vi "HandleTab.vi"(6 "Forward?":bool=TRUE, 8 "error in (no error)":errorcluster, 11 "TabbedControls":T1[](array[typedef])) -> (0 "error out":errorcluster, 3 "Discard?":bool)   [LabVIEW 2017, in "ContextHelpEditor.lvlib"]
uses:
  ContextHelpEditor.lvlib
  TabbedControl--cluster.ctl
  TabChange State--cluster.ctl
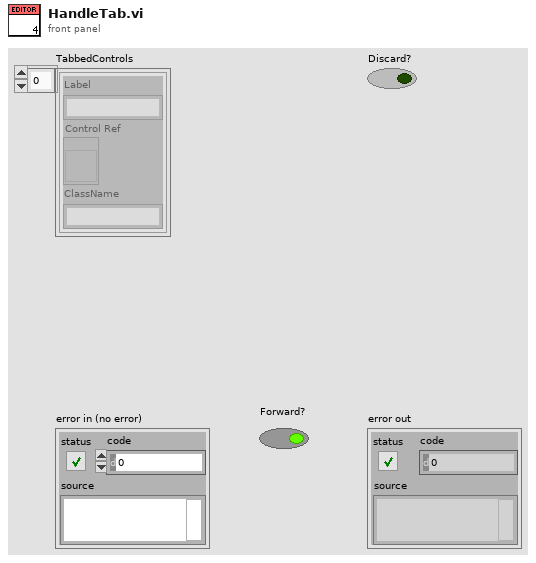
[diagram p1: front panel]
types:
  T1 = typedef "ContextHelpEditor.lvlib/TabbedControl--cluster.ctl" = cluster{"Label":string, "Control Ref":refnum<vi>, "ClassName":string}
  T2 = typedef "ContextHelpEditor.lvlib/TabChange State--cluster.ctl" = enum16{"CHECK_CURRENT_TYPE", "CHECK_PREVIOUS_TYPE", "CHECK_NEXT_TYPE", "CHECK_JUMP_INNER_MCLISTBOX", "JUMP_CURRENT_FW_MCLISTBOX", "JUMP_CURRENT_BACK_MCLISTBOX", "ACTIVATE_FIRST_ELEM_MCLISTBOX", "ACTIVATE_LAST_ELEM_MCLISTBOX", "ACTIVATE_NEXT_CONTROL", "ACTIVATE_PREV_CONTROL"}
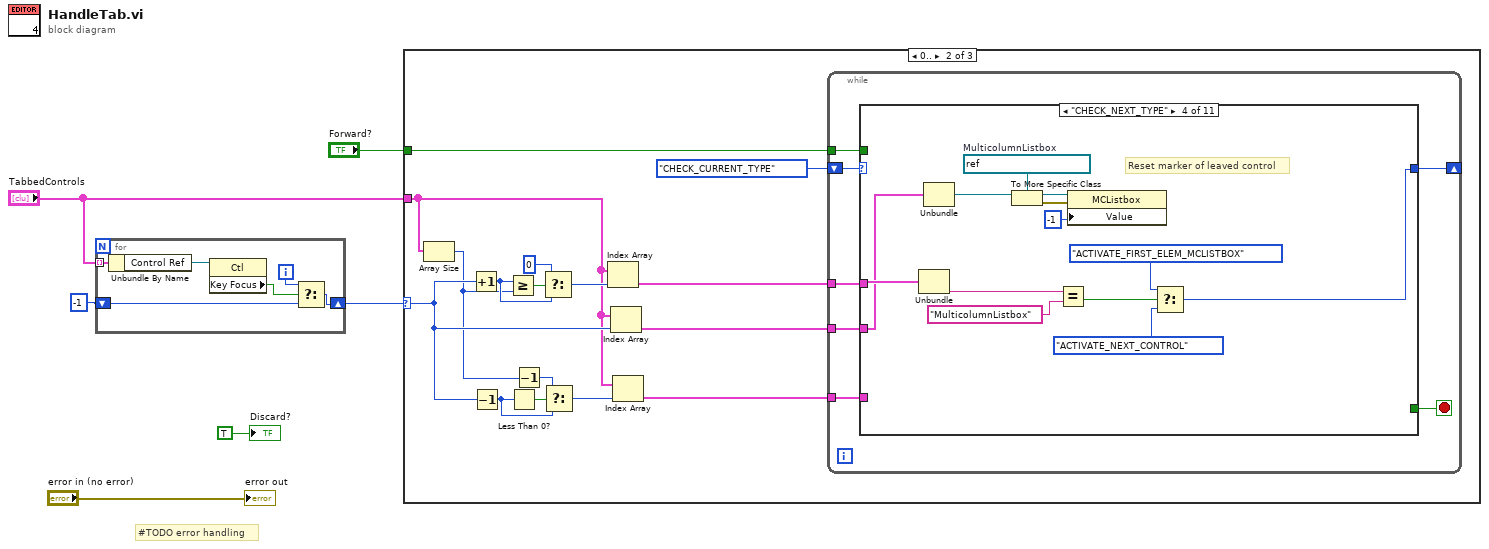
[diagram p0: block diagram]
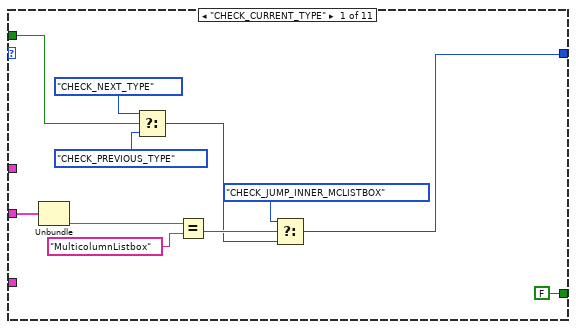
[diagram p3: hidden frame]
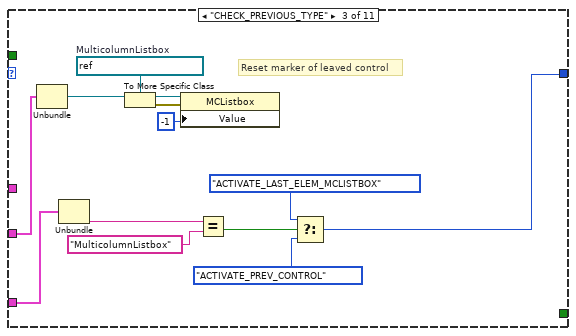
[diagram p5: hidden frame]
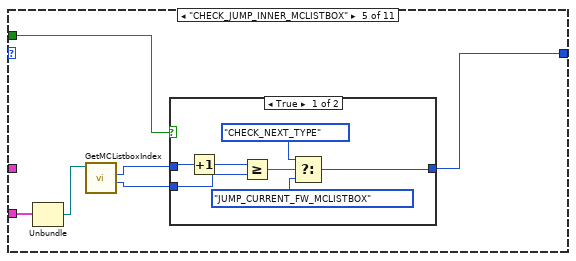
[diagram p6: hidden frame]
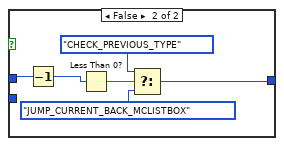
[diagram p7: hidden frame]
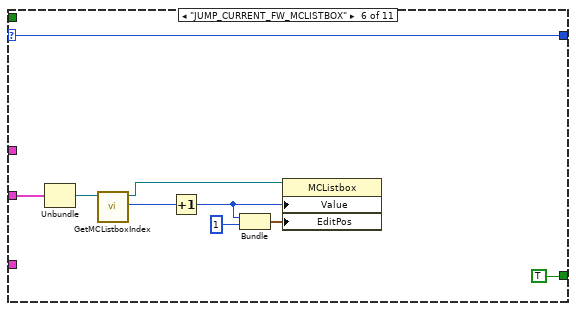
[diagram p8: hidden frame]
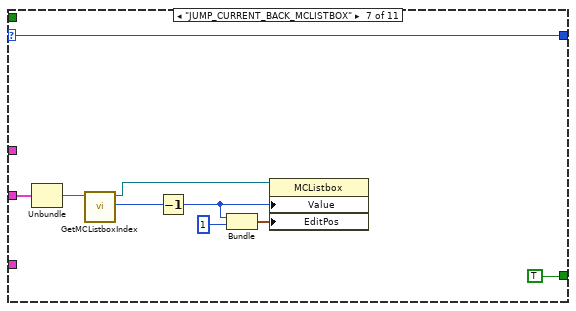
[diagram p9: hidden frame]
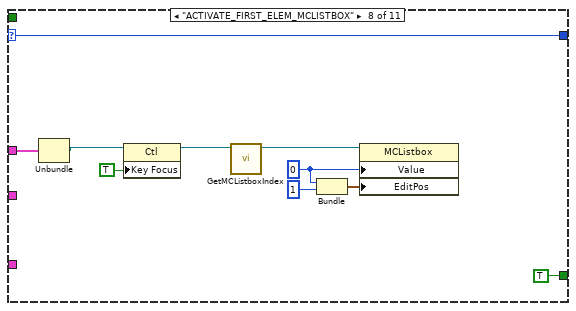
[diagram p10: hidden frame]
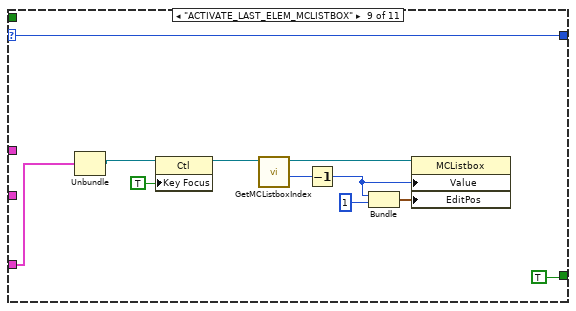
[diagram p11: hidden frame]
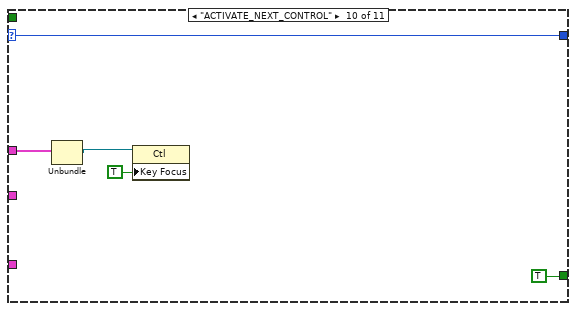
[diagram p12: hidden frame]
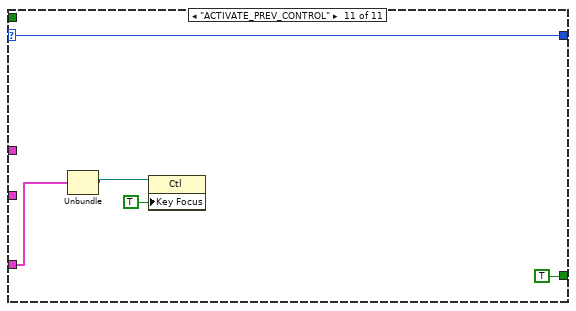
[diagram p13: hidden frame]
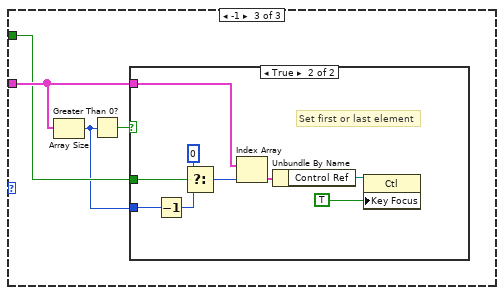
[diagram p14: hidden frame]
diagram:
  # "#TODO error handling"
  n1 = for {
    tunnel: "TabbedControls" -> [w12] mode=indexing
    shift-right: [w10] -> w3
    shift-left: -1 -> [w7]
    i -> [w8]
    n2 = Unbundle By Name(w12) -> ("Control Ref"=w11:refnum<vi>)
    n3 = property class="Ctl"(reference=w11) -> ("Key Focus"=w9:bool)  [unwired: 1 in, 2 out]
    n4 = Select(t=w8, s=w9, f=w7) -> (s? t:f=w10:i32)
  }
  n5 = case shown="0.." w3 {
    selector: w3 -> [_ w23 _]
    tunnel: "TabbedControls" -> [_ w19 w145]
    tunnel: "Forward?" -> [_ w16 w143]
    frame Default {
    }
    frame 0.. {
      n6 = Array Size(array=w19) -> (size(s)=w21:i32)
      n7 = Increment(x=w23) -> (x+1=w25:i32)
      n8 = Decrement(x=w23) -> (x-1=w22:i32)
      n9 = Greater Or Equal?(x=w25, y=w21) -> (x >= y?=w28:bool)
      n10 = Less Than 0?(x=w22) -> (x < 0?=w24:bool)
      n11 = Decrement(x=w21) -> (x-1=w20:i32)
      n12 = Select(t=0, s=w28, f=w25) -> (s? t:f=w26:i32)
      n13 = Select(t=w20, s=w24, f=w22) -> (s? t:f=w18:i32)
      n14 = Index Array(array=w19, index=w26) -> (element=w15:T1)
      n15 = Index Array(array=w19, index=w23) -> (element=w14:T1)
      n16 = Index Array(array=w19, index=w18) -> (element=w13:T1)
      n17 = while {
        shift-right: [w34] -> _
        shift-left: TabChange_State--cluster."CHECK_CURRENT_TYPE" -> [w35]
        tunnel: w16 -> [w33]
        tunnel: w15 -> [w31]
        tunnel: w14 -> [w30]
        tunnel: w13 -> [w29]
        stop <- w32 stop-if-true
        n18 = case shown="\"CHECK_NEXT_TYPE\"" w35 {
          selector: w35 -> [_ w47 _ _ _ w93 w102 w113 w121 w132 w137]
          tunnel: [w37 w47 w54 w67 w76 w93 w102 w113 w121 w132 w137] -> w34
          tunnel: w33 -> [w42 _ _ _ w77 _ _ _ _ _ _]
          tunnel: [FALSE _ _ _ _ TRUE TRUE TRUE TRUE TRUE TRUE] -> w32
          tunnel: w31 -> [_ _ _ w70 _ _ _ w117 _ w134 _]
          tunnel: w30 -> [w45 _ w51 w61 w79 w100 w104 _ _ _ _]
          tunnel: w29 -> [_ _ w55 _ _ _ _ _ w127 _ w139]
          frame "CHECK_CURRENT_TYPE" {
            n19 = Unbundle(w45) -> ("ClassName"=w44:string)  [unwired: 2 out]
            n20 = Select(t=TabChange_State--cluster."CHECK_NEXT_TYPE", s=w42, f=TabChange_State--cluster."CHECK_PREVIOUS_TYPE") -> (s? t:f=w38:T2)
            n21 = Equal?(x=w44, y="MulticolumnListbox") -> (x = y?=w39:bool)
            n22 = Select(t=TabChange_State--cluster."CHECK_JUMP_INNER_MCLISTBOX", s=w39, f=w38) -> (s? t:f=w37:T2)
          }
          frame Default {
          }
          frame "CHECK_PREVIOUS_TYPE" {
            w48 = refnum<vi> refnum  # MulticolumnListbox
            # "Reset marker of leaved control"
            n23 = Unbundle(w51) -> ("Control Ref"=w52:refnum<vi>)  [unwired: 2 out]
            n24 = Unbundle(w55) -> ("ClassName"=w60:string)  [unwired: 2 out]
            n25 = To More Specific Class(target class=w48, reference=w52) -> (specific class reference=w49:refnum<vi>, error out=w50:errorcluster)  [unwired: 1 in]
            n26 = property class="MCListbox"(reference=w49, error in=w50, "Value"=-1) -> ()  [unwired: 2 out]
            n27 = Equal?(x=w60, y="MulticolumnListbox") -> (x = y?=w58:bool)
            n28 = Select(t=TabChange_State--cluster."ACTIVATE_LAST_ELEM_MCLISTBOX", s=w58, f=TabChange_State--cluster."ACTIVATE_PREV_CONTROL") -> (s? t:f=w54:T2)
          }
          frame "CHECK_NEXT_TYPE" {
            w62 = refnum<vi> refnum  # MulticolumnListbox
            # "Reset marker of leaved control"
            n29 = Unbundle(w70) -> ("ClassName"=w73:string)  [unwired: 2 out]
            n30 = Unbundle(w61) -> ("Control Ref"=w65:refnum<vi>)  [unwired: 2 out]
            n31 = To More Specific Class(target class=w62, reference=w65) -> (specific class reference=w63:refnum<vi>, error out=w64:errorcluster)  [unwired: 1 in]
            n32 = Equal?(x=w73, y="MulticolumnListbox") -> (x = y?=w71:bool)
            n33 = property class="MCListbox"(reference=w63, error in=w64, "Value"=-1) -> ()  [unwired: 2 out]
            n34 = Select(t=TabChange_State--cluster."ACTIVATE_FIRST_ELEM_MCLISTBOX", s=w71, f=TabChange_State--cluster."ACTIVATE_NEXT_CONTROL") -> (s? t:f=w67:T2)
          }
          frame "CHECK_JUMP_INNER_MCLISTBOX" {
            n35 = Unbundle(w79) -> ("Control Ref"=w78:refnum<vi>)  [unwired: 2 out]
            n36 = call "GetMCListboxIndex.vi"("Control in"=w78) -> ("Size"=w75:i32, "Index"=w74:i32)  [unwired: 7 in, 2 out]
            n37 = case shown="True" w77 {
              tunnel: w75 -> [w84 _]
              tunnel: w74 -> [w83 w91]
              tunnel: [w81 w88] -> w76
              frame True {
                n38 = Increment(x=w83) -> (x+1=w86:i32)
                n39 = Greater Or Equal?(x=w86, y=w84) -> (x >= y?=w85:bool)
                n40 = Select(t=TabChange_State--cluster."CHECK_NEXT_TYPE", s=w85, f=TabChange_State--cluster."JUMP_CURRENT_FW_MCLISTBOX") -> (s? t:f=w81:T2)
              }
              frame False {
                n41 = Decrement(x=w91) -> (x-1=w89:i32)
                n42 = Less Than 0?(x=w89) -> (x < 0?=w92:bool)
                n43 = Select(t=TabChange_State--cluster."CHECK_PREVIOUS_TYPE", s=w92, f=TabChange_State--cluster."JUMP_CURRENT_BACK_MCLISTBOX") -> (s? t:f=w88:T2)
              }
            }
          }
          frame "JUMP_CURRENT_FW_MCLISTBOX" {
            n44 = Unbundle(w100) -> ("Control Ref"=w101:refnum<vi>)  [unwired: 2 out]
            n45 = call "GetMCListboxIndex.vi"("Control in"=w101) -> ("Index"=w99:i32, "MCListbox out"=w95:refnum<vi>)  [unwired: 7 in, 2 out]
            n46 = Increment(x=w99) -> (x+1=w96:i32)
            n47 = Bundle(w96, "index"=1) -> (w97:cluster{i32, "index":i32})  [unwired: 1 in]
            n48 = property class="MCListbox"(reference=w95, "Value"=w96, "EditPos"=w97) -> ()  [unwired: 1 in, 2 out]
          }
          frame "JUMP_CURRENT_BACK_MCLISTBOX" {
            n49 = Unbundle(w104) -> ("Control Ref"=w110:refnum<vi>)  [unwired: 2 out]
            n50 = call "GetMCListboxIndex.vi"("Control in"=w110) -> ("Index"=w109:i32, "MCListbox out"=w105:refnum<vi>)  [unwired: 7 in, 2 out]
            n51 = Decrement(x=w109) -> (x-1=w106:i32)
            n52 = Bundle(w106, "index"=1) -> (w107:cluster{i32, "index":i32})  [unwired: 1 in]
            n53 = property class="MCListbox"(reference=w105, "Value"=w106, "EditPos"=w107) -> ()  [unwired: 1 in, 2 out]
          }
          frame "ACTIVATE_FIRST_ELEM_MCLISTBOX" {
            w115 = 0 ("index")
            n54 = Unbundle(w117) -> ("Control Ref"=w116:refnum<vi>)  [unwired: 2 out]
            n55 = property class="Ctl"(reference=w116, "Key Focus"=TRUE) -> (reference out=w112:refnum<vi>)  [unwired: 1 in, 1 out]
            n56 = call "GetMCListboxIndex.vi"("Control in"=w112) -> ("MCListbox out"=w118:refnum<vi>)  [unwired: 7 in, 3 out]
            n57 = Bundle("index"=w115, "index"=1) -> (w119:cluster{"index":i32, "index":i32})  [unwired: 1 in]
            n58 = property class="MCListbox"(reference=w118, "Value"=w115, "EditPos"=w119) -> ()  [unwired: 1 in, 2 out]
          }
          frame "ACTIVATE_LAST_ELEM_MCLISTBOX" {
            n59 = Unbundle(w127) -> ("Control Ref"=w128:refnum<vi>)  [unwired: 2 out]
            n60 = property class="Ctl"(reference=w128, "Key Focus"=TRUE) -> (reference out=w123:refnum<vi>)  [unwired: 1 in, 1 out]
            n61 = call "GetMCListboxIndex.vi"("Control in"=w123) -> ("Size"=w125:i32, "MCListbox out"=w129:refnum<vi>)  [unwired: 7 in, 2 out]
            n62 = Decrement(x=w125) -> (x-1=w126:i32)
            n63 = Bundle(w126, "index"=1) -> (w130:cluster{i32, "index":i32})  [unwired: 1 in]
            n64 = property class="MCListbox"(reference=w129, "Value"=w126, "EditPos"=w130) -> ()  [unwired: 1 in, 2 out]
          }
          frame "ACTIVATE_NEXT_CONTROL" {
            n65 = Unbundle(w134) -> ("Control Ref"=w136:refnum<vi>)  [unwired: 2 out]
            n66 = property class="Ctl"(reference=w136, "Key Focus"=TRUE) -> ()  [unwired: 1 in, 2 out]
          }
          frame "ACTIVATE_PREV_CONTROL" {
            n67 = Unbundle(w139) -> ("Control Ref"=w141:refnum<vi>)  [unwired: 2 out]
            n68 = property class="Ctl"(reference=w141, "Key Focus"=TRUE) -> ()  [unwired: 1 in, 2 out]
          }
        }
      }
    }
    frame -1 {
      n69 = Array Size(array=w145) -> (size(s)=w142:i32)
      n70 = Greater Than 0?(x=w142) -> (x > 0?=w144:bool)
      n71 = case shown="True" w144 {
        tunnel: w145 -> [_ w153]
        tunnel: w143 -> [_ w150]
        tunnel: w142 -> [_ w146]
        frame False {
        }
        frame True {
          # "Set first or last element"
          n72 = Decrement(x=w146) -> (x-1=w147:i32)
          n73 = Select(t=0, s=w150, f=w147) -> (s? t:f=w148:i32)
          n74 = Index Array(array=w153, index=w148) -> (element=w152:T1)
          n75 = Unbundle By Name(w152) -> ("Control Ref"=w151:refnum<vi>)
          n76 = property class="Ctl"(reference=w151, "Key Focus"=TRUE) -> ()  [unwired: 1 in, 2 out]
        }
      }
    }
  }
  "Discard?" <- TRUE
  "error out" <- "error in (no error)"
